vi "VISA Configure Serial Port (Serial Instr).vi"(0 "VISA resource name":refnum<visa-resource-name>, 1 "timeout (10sec)":u32=10000, 2 "termination char\n(0xA = '\\n' = LF)":u8=10 format="%.0x", 3 "Enable Termination\nChar (T)":bool=TRUE, 5 "baud rate (9600)":u32=9600, 7 "data bits (8)":u16=8 min=5 max=8 step=1, 9 "parity (0:none)":enum16{"None", "Odd", "Even", "Mark", "Space"}(ring), 11 "error in (no error)":errorcluster, 12 "stop bits (10: 1 bit)":u16(ring)=10 items=["1.0"=10, "1.5"=15, "2.0"=20], 13 "flow control (0:none)":u16(ring) items=["None", "XON/XOFF", "RTS/CTS", "XON/XOFF & RTS/CTS", "DTR/DSR", "XON/XOFF & DTR/DSR"]) -> (4 "VISA resource name out":refnum<visa-resource-name>, 15 "error out":errorcluster)   [LabVIEW 2022 SP3]
doc: "Initializes the serial port specified by <B>VISA resource name</B> to the specified settings. Wire data to the <B>VISA resource name</B> input to determine the polymorphic instance to use or manually select the instance."
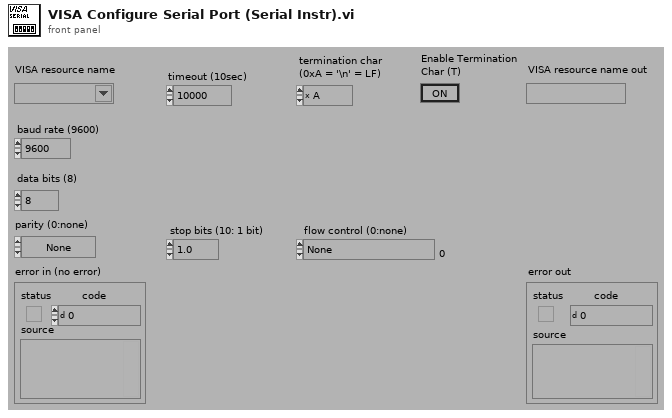
[diagram p1: front panel]
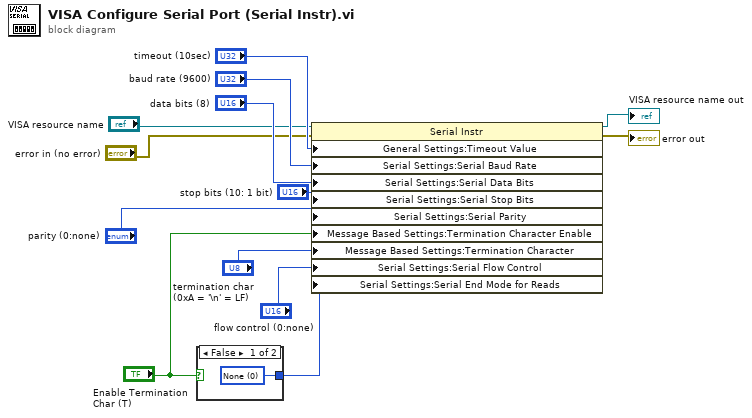
[diagram p0: block diagram]
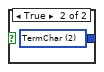
[diagram p2: hidden frame]
diagram:
  n1 = case shown="False" "Enable Termination\nChar (T)" {
    tunnel: [w14 w15] -> w3
    frame False {
      w14 = u16 0 items=["None", "LastBit", "TermChar"] ("Serial Settings:Serial End Mode for Reads")
    }
    frame True {
      w15 = u16 2 items=["None", "LastBit", "TermChar"] ("Serial Settings:Serial End Mode for Reads")
    }
  }
  n2 = property class="Serial Instr"(reference="VISA resource name", error in="error in (no error)", "General Settings:Timeout Value"="timeout (10sec)", "Serial Settings:Serial Baud Rate"="baud rate (9600)", "Serial Settings:Serial Data Bits"="data bits (8)", "Serial Settings:Serial Stop Bits"="stop bits (10: 1 bit)", "Serial Settings:Serial Parity"="parity (0:none)", "Message Based Settings:Termination Character Enable"="Enable Termination\nChar (T)", "Message Based Settings:Termination Character"="termination char\n(0xA = '\\n' = LF)", "Serial Settings:Serial Flow Control"="flow control (0:none)", "Serial Settings:Serial End Mode for Reads"=w3) -> (reference out=→"VISA resource name out":refnum<visa-resource-name>, error out=→"error out":errorcluster)
